vi "Stop Core.vi"(10 "final error code":i32, 11 "Actor_Scope in":refnum<class "Actor_Scope.lvclass">) -> (3 "Actor_Scope out":refnum<class "Actor_Scope.lvclass">)   [LabVIEW 2020, in "Actor_Scope.lvlib" / "Actor_Scope.lvclass"]
doc: "(<B>Filename</B>: Actor Framework.lvlib:Actor.lvclass:Stop Core.vi)\n\nDefines what the actor does before it stops. Use the <B>final error code</B> input to determine whether the actor shut down in response to an error.\n\nBy default, this method passes the Stop message along to all auto-stop nested actors. A descendant class may override this method to define additional behavior, such as shutting down any processes the actor initiated in its override of the Actor Core method."
uses:
  Actor_Scope.lvclass
  Actor_Scope.lvclass/Actor_Scope.ctl
  <vilib>/ActorFramework/Actor/Actor.lvclass
  <instrlib>/Agilent 8000 Series/Agilent 8000 Series.lvlib
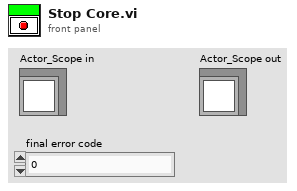
[diagram p1: front panel]
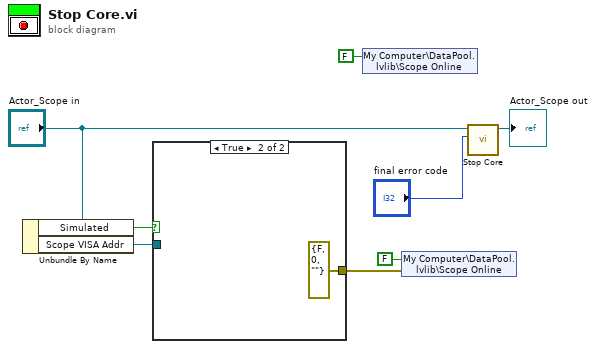
[diagram p0: block diagram]
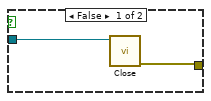
[diagram p2: hidden frame]
diagram:
  n1 = Unbundle By Name("Actor_Scope in") -> ("Simulated"=w4:bool, "Scope VISA Addr"=w3:refnum<visa-resource-name>)
  n2 = case shown="True" w4 {
    tunnel: w3 -> [w10 _]
    tunnel: [w9 errorcluster {"status"=FALSE, "code"=0, "source"=""} ("error out")] -> w2
    frame False {
      n3 = call <instrlib>:"Close.vi"("VISA resource name"=w10) -> ("error out"=w9:errorcluster)  [unwired: 10 in]
    }
    frame True {
    }
  }
  n4 = shared-variable "My Computer\\DataPool.lvlib\\Scope Online"(FALSE ("AFG Online")) -> ()  [unwired: 1 in, 1 out]
  n5 = shared-variable "My Computer\\DataPool.lvlib\\Scope Online"(FALSE ("Scope Online"), error in=w2) -> ()  [unwired: 1 out]
  n6 = call-parent "Stop Core.vi"("final error code"="final error code", "Actor in"="Actor_Scope in") -> ("Actor out"=→"Actor_Scope out":refnum<class "Actor_Scope.lvclass">)  [unwired: 9 in]
